vi "RunTest.vi"(8 "error in (no error)":errorcluster, 11 "Prueba01 in":refnum<class "Prueba01.lvclass">) -> (0 "error out":errorcluster, 2 "resultado":string, 3 "Prueba01 out":refnum<class "Prueba01.lvclass">)   [LabVIEW 2019, in "Prueba01.lvclass"]
uses:
  Prueba01.lvclass
  Controles/MessageP01.ctl
  Controles/EstadosP01.ctl
  Prueba01.lvclass/Prueba01.ctl
  RerenceAllControlsToolkit/_get control reference by name.vi
  RerenceAllControlsToolkit/_get mutiple control reference by name.vi
  Instrumento/CNT90/CNT90.lvclass
  Instrumento/Keithley2002/Keithley2002.lvclass
  Instrumento/DS360/DS360.lvclass
panel:
  in  "Tab Control":enum32{"externo", "interno"}(tab)
  out "max_tol_ajuste_ext":dbl format="%.1f"
  out "nivel_ref":dbl
  in  "generar":bool
  out "frec_ref":dbl
  out "cumple":bool
  out "no_cumple":bool
  out "frecuencia":dbl format="%.1f"
  out "nivel":dbl
  in  "señal_antes_ajuste":dbl format="%.1f"
  out "error_ext":dbl
  out "inc_expand_ext":dbl
  in  "seguir_ext":bool
  out "voltaje":dbl
  out "frecuencia 2":dbl
  out "tipo generador":string
  out "max_tol_ajuste_int":dbl
  out "Nivel_interno":dbl
  out "frecuencia_int":dbl
  out "cumple_int":bool
  out "no_cumple_int":bool
  out "frec_ref_int":dbl
  out "nivel_ref_int":dbl
  in  "señal_antes_ajuste_int":dbl
  out "error_ext_int":dbl
  out "inc_extend_int":dbl
  in  "seguir_int":bool
  out "tipo gen_int":string
  # "Elección Señal de Referencia \nsegún marca y modelo de sonómetro"
  # "Cumple"
  # "No Cumple"
  # "Máxima Tolerancia de Ajuste"
  # "Frecuencia"
  # "Nivel"
  # "Frecuencia Señal de Referencia [Hz]"
  # "Nivel de Señal de Referencia [dB] (a)"
  # "Nivel de señal medida antes de ajuste [dB] (b)"
  # "Error [dB]"
  # "Incertidumbre Expandida ± [dB] (k=2)"
  # "1. Indicación a la frecuencia de comprobación. IEC 61672-3: 2006 Cláusula 9"
  # "Monitoreo"
  # "Frecuencia"
  # "Hz"
  # "Voltaje"
  # "V"
  # "Elección Señal de Referencia \nsegún marca y modelo de sonómetro"
  # "Máxima Tolerancia de ajuste"
  # "Cumple"
  # "No Cumple"
  # "Frecuencia"
  # "Nivel"
  # "Frecuencia Señal de Referencia [Hz]"
  # "Nivel de Señal de Referencia [dB] (a)"
  # "Nivel de señal medida antes de ajuste [dB] (b)"
  # "Error [dB]"
  # "Incertidumbre Expandida ± [dB] (k=2)"
  # "1. Indicación a la frecuencia de comprobación. IEC 61672-3: 2006 Cláusula 9"
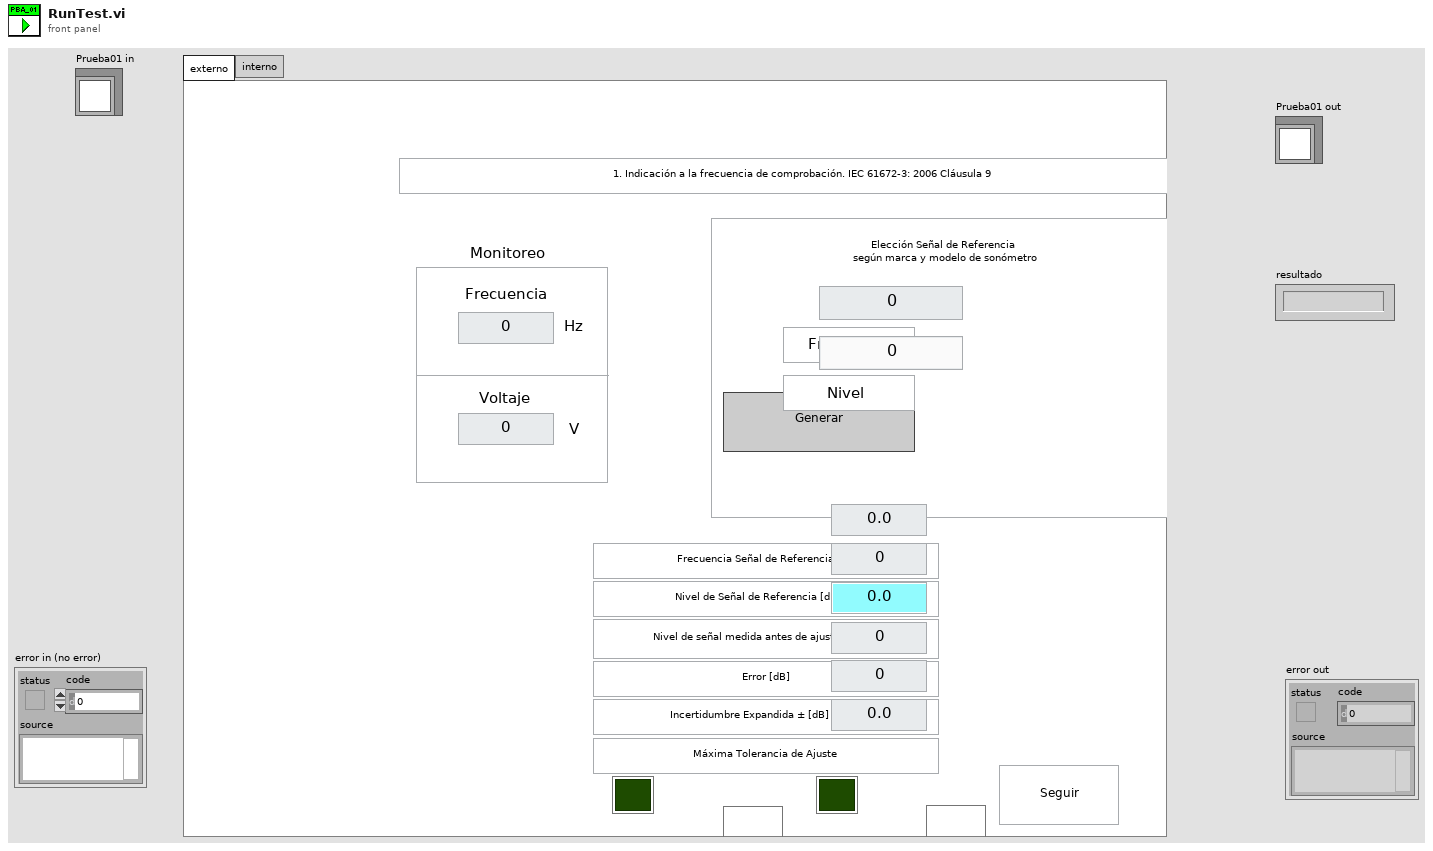
[diagram p1: front panel]
types:
  T1 = typedef "Prueba01.lvclass/EstadosP01.ctl" = enum16{"Inicio", "LeeArchivoConf", "LeeTipoGenerador", "inicio_ext", "inicio_int", "leer_BD", "leer_BD_int", "FrecAmpGEN_ext", "iniciarGEN_ext", "monitoreo", "detenerGEN_ext", "cumplimiento_ext", "cumplimiento_int", "Confirmar Salir", "salir"}
  T2 = typedef "Prueba01.lvclass/MessageP01.ctl" = cluster{"Estados":T1, "Data":variant}
  T3 = enum8{"Enabled", "Disabled", "Disabled and Grayed Out"}
  T4 = cluster{"ControlName":string, "ControlReference":refnum<vi>}[]
  T5 = typedef "Prueba01.lvclass/BD_P01.ctl" = cluster{"frec_ref":dbl, "nivel_presion_ref":dbl, "max_tolerancia_aju":dbl, "inc_expand_ext":dbl, "vol_enviado_CAM":dbl}
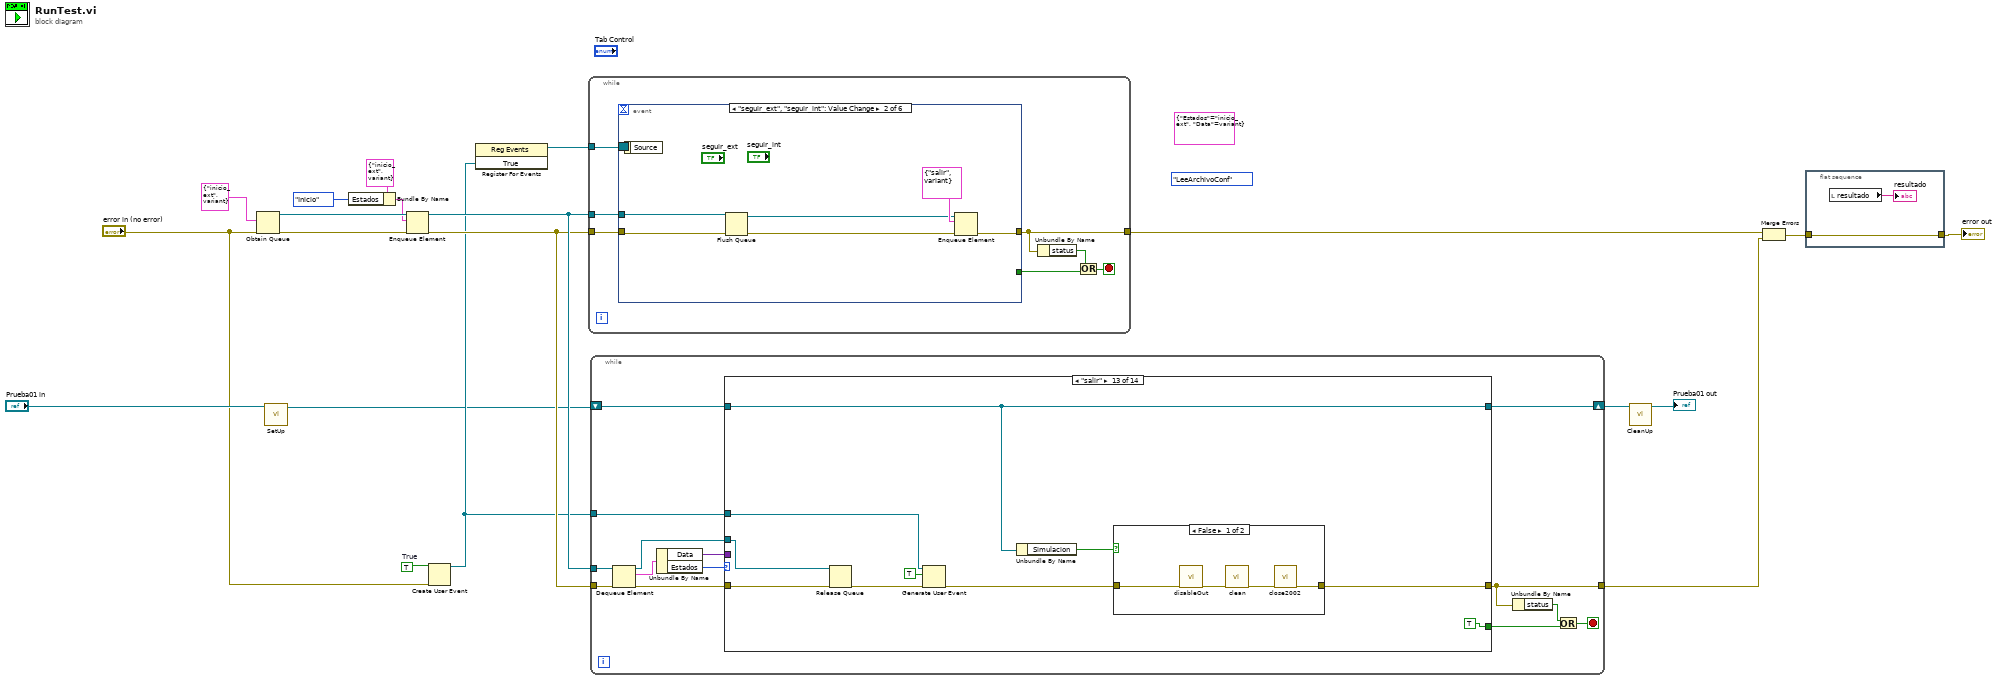
[diagram p0: block diagram]
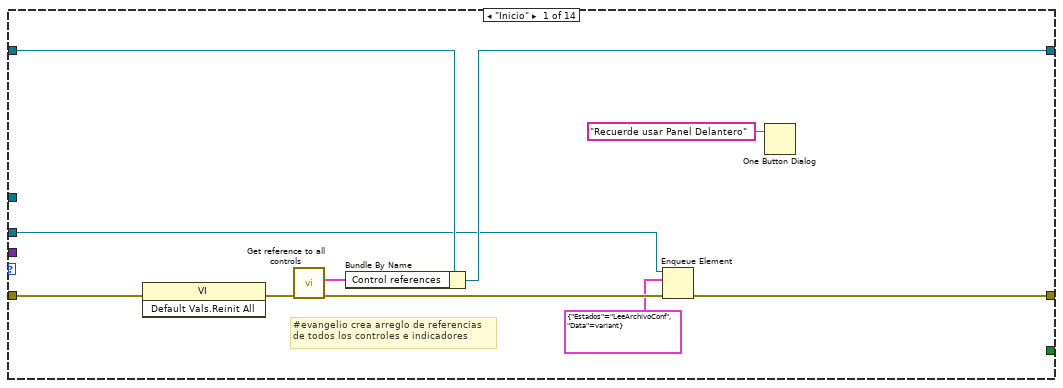
[diagram p2: hidden frame]
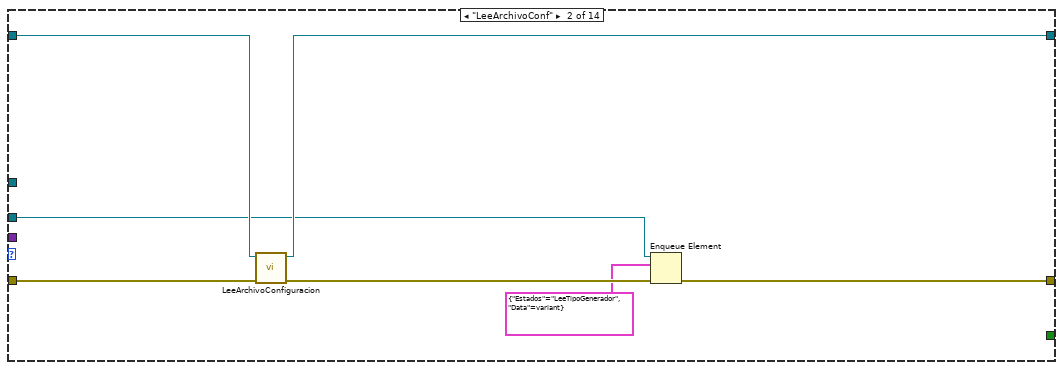
[diagram p3: hidden frame]
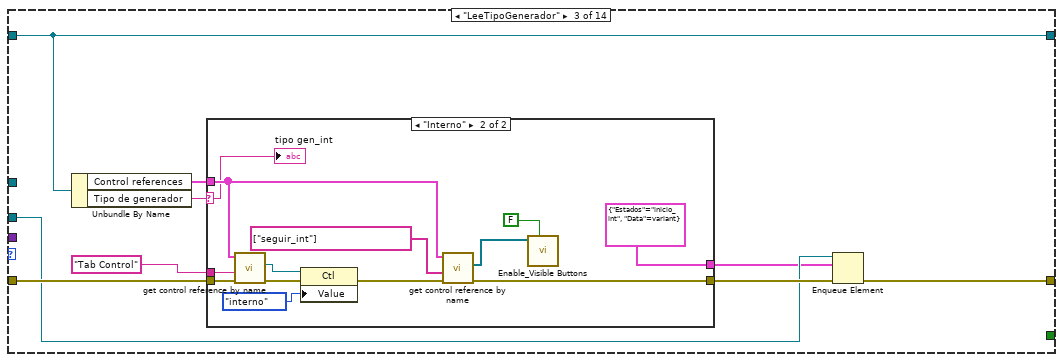
[diagram p4: hidden frame]
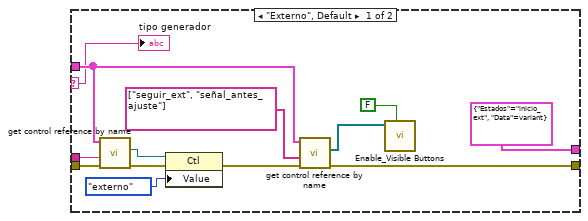
[diagram p5: hidden frame]
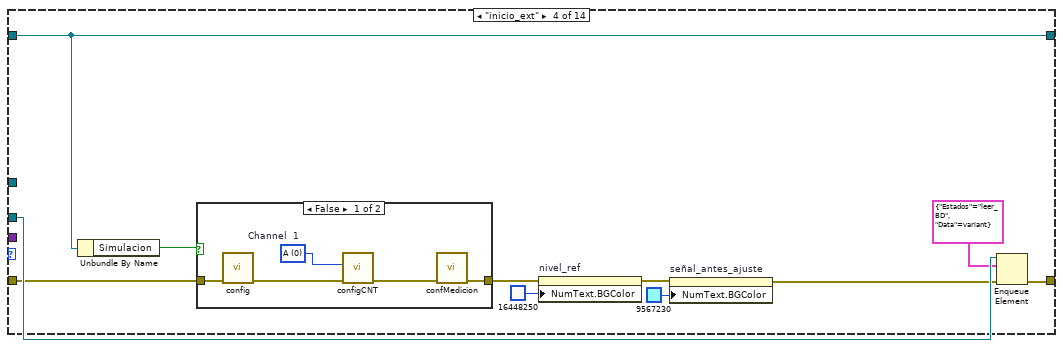
[diagram p6: hidden frame]
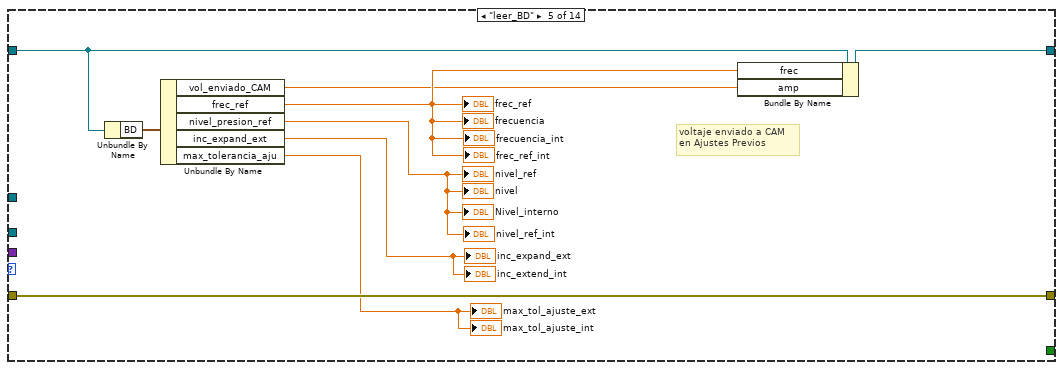
[diagram p8: hidden frame]
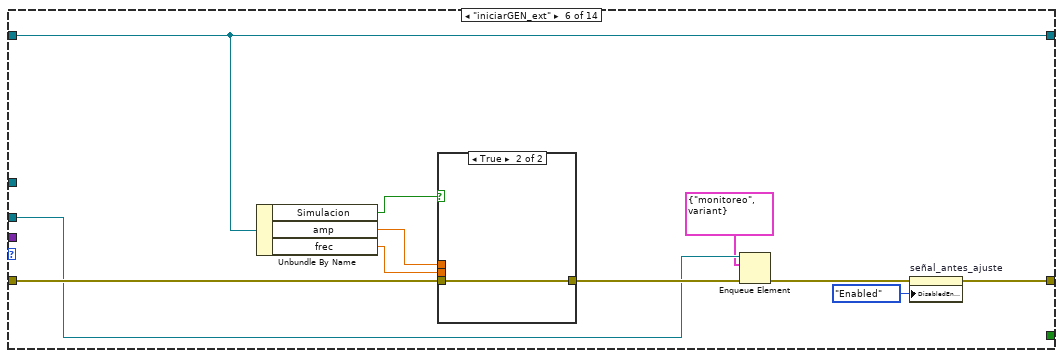
[diagram p9: hidden frame]
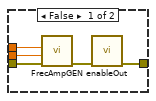
[diagram p10: hidden frame]
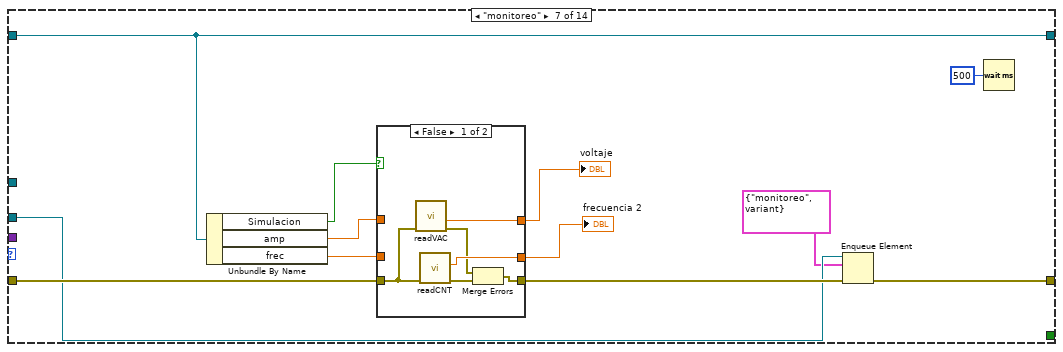
[diagram p11: hidden frame]
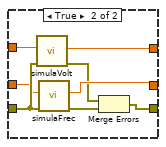
[diagram p12: hidden frame]
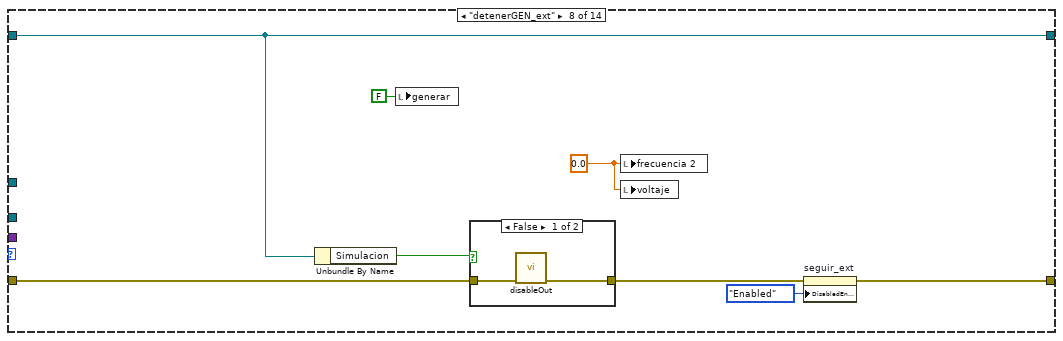
[diagram p13: hidden frame]
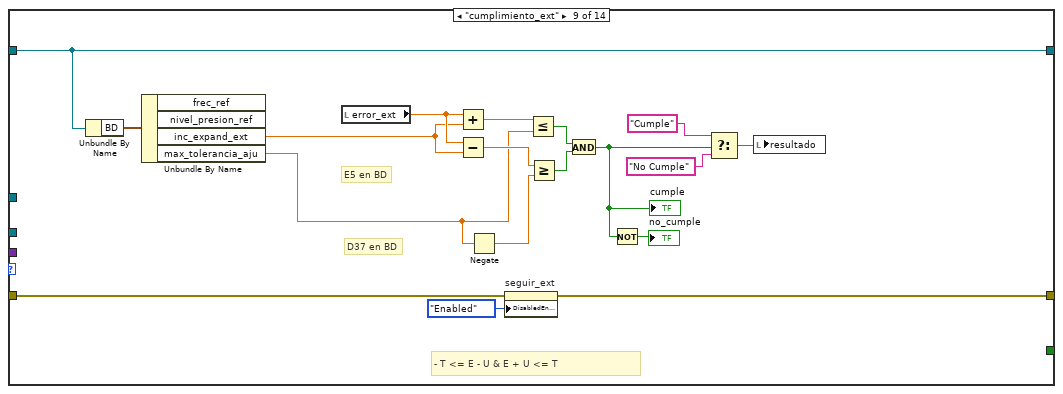
[diagram p15: hidden frame]
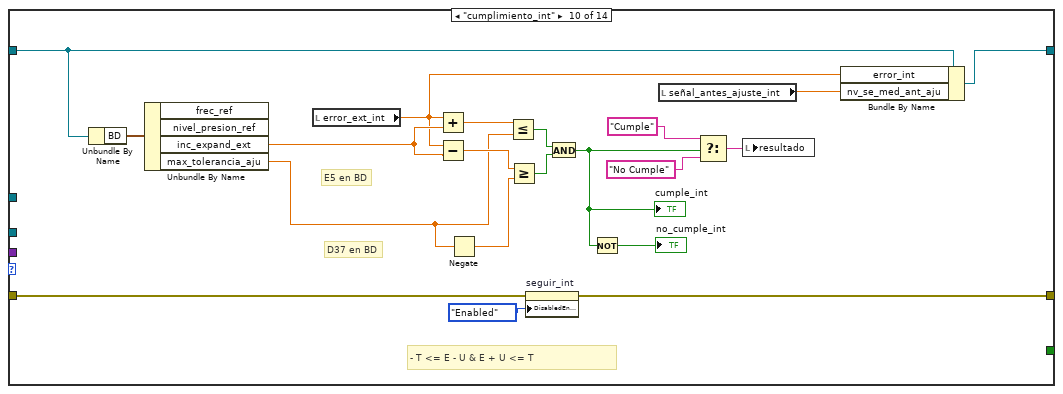
[diagram p16: hidden frame]
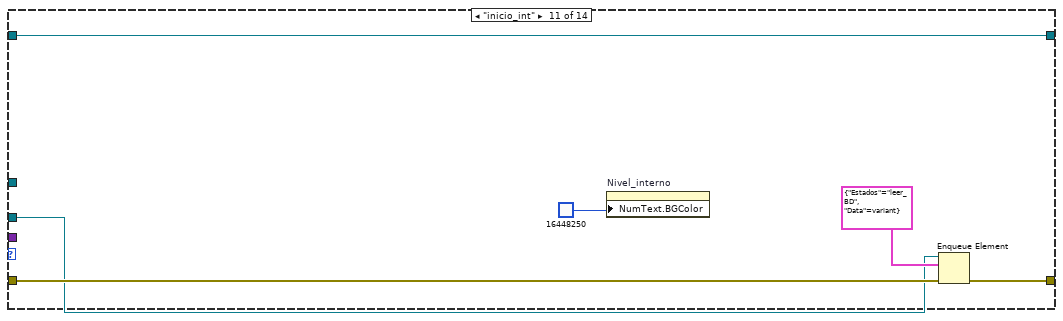
[diagram p17: hidden frame]
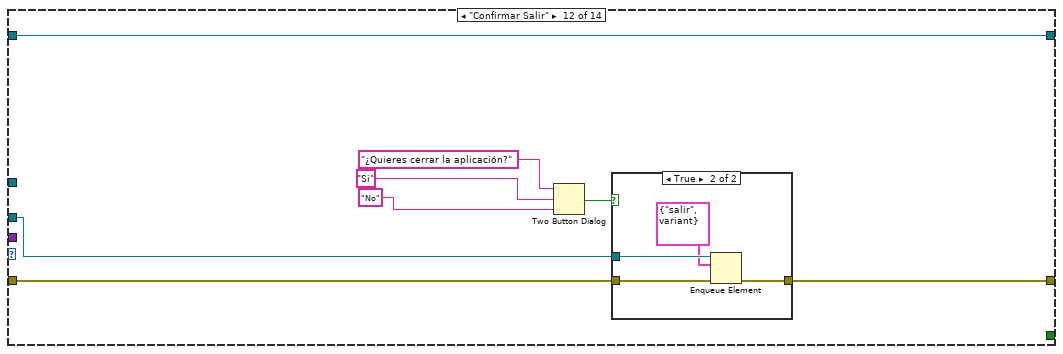
[diagram p18: hidden frame]
diagram:
  w5 = TRUE  # True
  (unwired) EstadosP01."LeeArchivoConf" ("Estados")
  (unwired) T2 {"Estados"=enum."inicio_ext", "Data"=variant}
  n1 = Obtain Queue(element data type=T2 {"Estados"=enum."inicio_ext", "Data"=variant}, error in (no error)="error in (no error)") -> (queue out=w19:refnum<queue>, error out=w18:errorcluster)  [unwired: 3 in, 1 out]
  n2 = call-dynamic "SetUp.vi"("Prueba01 in"="Prueba01 in") -> ("Prueba01 out"=w1:refnum<class "Prueba01.lvclass">)  [unwired: 9 in, 1 out]
  n3 = Bundle By Name(cluster=T2 {"Estados"=enum."inicio_ext", "Data"=variant}, "Estados"=EstadosP01."Inicio") -> (w11:T2)
  n4 = Enqueue Element(queue=w19, element=w11, error in (no error)=w18) -> (queue out=w16:refnum<queue>, error out=w15:errorcluster)  [unwired: 1 in, 1 out]
  n5 = Create User Event(user event datatype=w5, error in="error in (no error)") -> (user event=w2:refnum<user-event>)  [unwired: 1 out]
  n6 = register-events(w2) -> (reference out=w4:refnum<event-registration>)  [unwired: 2 in, 1 out]
  n7 = while {
    tunnel: w16 -> [w26]
    tunnel: w15 -> [w27]
    tunnel: [w24] -> w10
    tunnel: w4 -> [w25]
    stop <- w23 stop-if-true
    n8 = event shown="[1] \"seguir_ext\", \"seguir_int\": Value Change" {
      selector: w25 -> [_ _ _ _ _ _]
      dyn-events: _ -> [_ _ _ _ _ _]
      timeout: _ -> [_ _ _ _ _ _]
      tunnel: w27 -> [w31 w40 w41 w51 w57 w64]
      tunnel: w26 -> [w28 w36 _ w44 w54 w65]
      tunnel: [w30 w39 w41 w50 w55 w63] -> w24
      tunnel: [_ _ TRUE _ _ _] -> w21
      event "señal_antes_ajuste": Value Change {
        n9 = event-data() -> ("NewVal"=w33:dbl)  [unwired: 1 in]
        n10 = local read "nivel"() -> (w32:dbl)
        n11 = Subtract(x=w33, y=w32) -> (x-y=→"error_ext":dbl)
        n12 = Enqueue Element(queue=w28, element=T2 {"Estados"=enum."cumplimiento_ext", "Data"=variant}, error in (no error)=w31) -> (error out=w30:errorcluster)  [unwired: 1 in, 2 out]
      }
      event "seguir_ext", "seguir_int": Value Change {
        n13 = event-data() -> ()  [unwired: 1 in, 1 out]
        n14 = Flush Queue(queue=w36, error in (no error)=w40) -> (queue out=w35:refnum<queue>, error out=w37:errorcluster)  [unwired: 1 out]
        n15 = Enqueue Element(queue=w35, element=T2 {"Estados"=enum."salir", "Data"=variant}, error in (no error)=w37) -> (error out=w39:errorcluster)  [unwired: 1 in, 2 out]
      }
      event User Event {
        n16 = event-data() -> ()  [unwired: 1 in, 5 out]
      }
      event "generar": Value Change {
        n17 = event-data() -> ("NewVal"=w48:bool)  [unwired: 1 in]
        n18 = Flush Queue(queue=w44, error in (no error)=w51) -> (queue out=w43:refnum<queue>, error out=w45:errorcluster)  [unwired: 1 out]
        n19 = Equal?(x=w48, y=TRUE) -> (x = y?=w46:bool)
        n20 = case shown="True" w46 {
          tunnel: [T2 {"Estados"=enum."detenerGEN_ext", "Data"=variant} ("element") T2 {"Estados"=enum."iniciarGEN_ext", "Data"=variant} ("element")] -> w49
          frame False {
          }
          frame True {
          }
        }
        n21 = Enqueue Element(queue=w43, element=w49, error in (no error)=w45) -> (error out=w50:errorcluster)  [unwired: 1 in, 2 out]
      }
      event "señal_antes_ajuste_int": Value Change {
        n22 = event-data() -> ("NewVal"=w58:dbl)  [unwired: 1 in]
        n23 = local read "nivel_ref_int"() -> (w59:dbl)
        n24 = Subtract(x=w58, y=w59) -> (x-y=→"error_ext_int":dbl)
        n25 = Enqueue Element(queue=w54, element=T2 {"Estados"=enum."cumplimiento_int", "Data"=variant}, error in (no error)=w57) -> (error out=w55:errorcluster)  [unwired: 1 in, 2 out]
      }
      event Panel Close? {
        n26 = event-data() -> ()  [unwired: 1 in, 1 out]
        n27 = Enqueue Element(queue=w65, element=T2 {"Estados"=enum."Confirmar Salir", "Data"=variant}, error in (no error)=w64) -> (error out=w63:errorcluster)  [unwired: 1 in, 2 out]
        n28 = event-data("Discard?"=TRUE) -> ()  [unwired: 1 in, 1 out]
      }
    }
    n29 = Unbundle By Name(w24) -> ("status"=w22:bool)
    n30 = Or(x=w22, y=w21) -> (x .or. y?=w23:bool)
  }
  n31 = while {
    tunnel: w16 -> [w79]
    tunnel: w15 -> [w78]
    tunnel: [w68] -> w9
    shift-right: [w67] -> w14
    shift-left: w1 -> [w69]
    tunnel: w2 -> [w66]
    stop <- w72 stop-if-true
    n32 = Dequeue Element(queue=w79, error in (no error)=w78) -> (queue out=w76:refnum<queue>, element=w77:T2, error out=w73:errorcluster)  [unwired: 1 in, 1 out]
    n33 = Unbundle By Name(w77) -> ("Data"=w74:variant, "Estados"=w75:T1)
    n34 = case shown="\"salir\"" w75 {
      tunnel: w76 -> [w82 w91 w98 w138 _ w162 w183 _ _ _ w250 w257 w277 _]
      tunnel: w74 -> [_ _ _ _ _ _ _ _ _ _ _ _ _ _]
      tunnel: w73 -> [w87 w96 w102 w136 w157 w168 w185 w208 w229 w235 w252 w259 w278 w285]
      tunnel: [w83 w92 w99 w139 w157 w159 w186 w202 w213 w234 w251 w258 w274 w285] -> w68
      tunnel: [_ _ _ _ _ _ _ _ _ _ _ _ TRUE _] -> w70
      tunnel: w69 -> [w85 w95 w100 w133 w155 w166 w180 w204 w216 w233 w255 w263 w273 w284]
      tunnel: [w84 w94 w100 w133 w156 w166 w180 w204 w216 w232 w255 w263 w273 w284] -> w67
      tunnel: w66 -> [_ _ _ _ _ _ _ _ _ _ _ _ w270 _]
      frame "Inicio" {
        # "#evangelio crea arreglo de referencias\nde todos los controles e indicadores"
        n35 = invoke class="VI" method="Default Vals.Reinit All"(error in=w87) -> (error out=w89:errorcluster)  [unwired: 2 in, 2 out]
        n36 = call "Get reference to all controls.vi"("error in (no error)"=w89) -> ("error out"=w86:errorcluster, "Control references"=w88:T4)  [unwired: 5 in]
        n37 = Bundle By Name(cluster=w85, "Control references"=w88) -> (w84:refnum<class "Prueba01.lvclass">)
        n38 = Enqueue Element(queue=w82, element=T2 {"Estados"=enum."LeeArchivoConf", "Data"=variant}, error in (no error)=w86) -> (error out=w83:errorcluster)  [unwired: 1 in, 2 out]
        n39 = One Button Dialog(message="Recuerde usar Panel Delantero") -> ()  [unwired: 1 in, 1 out]
      }
      frame "LeeArchivoConf" {
        n40 = call "LeeArchivoConfiguracion.vi"("error in (no error)"=w96, "Prueba01 in"=w95) -> ("error out"=w93:errorcluster, "Prueba01 out"=w94:refnum<class "Prueba01.lvclass">)  [unwired: 8 in]
        n41 = Enqueue Element(queue=w91, element=T2 {"Estados"=enum."LeeTipoGenerador", "Data"=variant}, error in (no error)=w93) -> (error out=w92:errorcluster)  [unwired: 1 in, 2 out]
      }
      frame "LeeTipoGenerador" {
        n42 = Unbundle By Name(w100) -> ("Control references"=w104:T4, "Tipo de generador"=w105:string)
        n43 = case shown="\"Interno\"" w105 {
          selector: w105 -> [w109 w122]
          tunnel: w102 -> [w118 w131]
          tunnel: w104 -> [w113 w126]
          tunnel: "Tab Control" -> [w117 w130]
          tunnel: [w111 w124] -> w101
          tunnel: [T2 {"Estados"=enum."inicio_ext", "Data"=variant} ("element") T2 {"Estados"=enum."inicio_int", "Data"=variant} ("element")] -> w97
          frame "Externo", Default {
            n44 = call-poly "get control reference by name.vi"("error in (no error)"=w118, "Control name"=w117, "Control references"=w113) -> ("error out"=w115:errorcluster, "Ctl Refnum"=w116:refnum<vi>)  [unwired: 3 in]
            n45 = property class="Ctl"(reference=w116, error in=w115, "Value"=enum32{"externo", "interno"}."externo" ("Tab Control")) -> (error out=w112:errorcluster)  [unwired: 1 out]
            n46 = call-poly "get control reference by name.vi"("error in (no error)"=w112, "Control names"=string[] ["seguir_ext", "señal_antes_ajuste"], "Control references"=w113) -> ("error out"=w111:errorcluster, "References"=w106:refnum<vi>[])  [unwired: 3 in]
            n47 = call "Enable_Visible Buttons.vi"("Enable? (T)"=FALSE, "Controls Ref Array"=w106) -> ()  [unwired: 10 in]
            "tipo generador" <- w109
          }
          frame "Interno" {
            n48 = call-poly "get control reference by name.vi"("error in (no error)"=w131, "Control name"=w130, "Control references"=w126) -> ("error out"=w128:errorcluster, "Ctl Refnum"=w129:refnum<vi>)  [unwired: 3 in]
            n49 = property class="Ctl"(reference=w129, error in=w128, "Value"=enum32{"externo", "interno"}."interno" ("Tab Control")) -> (error out=w125:errorcluster)  [unwired: 1 out]
            n50 = call-poly "get control reference by name.vi"("error in (no error)"=w125, "Control names"=string[] ["seguir_int"], "Control references"=w126) -> ("error out"=w124:errorcluster, "References"=w119:refnum<vi>[])  [unwired: 3 in]
            n51 = call "Enable_Visible Buttons.vi"("Enable? (T)"=FALSE, "Controls Ref Array"=w119) -> ()  [unwired: 10 in]
            "tipo gen_int" <- w122
          }
        }
        n52 = Enqueue Element(queue=w98, element=w97, error in (no error)=w101) -> (error out=w99:errorcluster)  [unwired: 1 in, 2 out]
      }
      frame "inicio_ext" {
        n53 = Unbundle By Name(w133) -> ("Simulacion"=w132:bool)
        n54 = case shown="False" w132 {
          tunnel: w136 -> [w146 w148]
          tunnel: [w143 w148] -> w135
          frame False {
            w145 = 0 items=["A", "B"]  # Channel  1
            n55 = call "config.vi"("error in (no error)"=w146) -> ("error out"=w147:errorcluster)  [unwired: 9 in, 1 out]
            n56 = call "configCNT.vi"("error in (no error)"=w147, "Channel  1"=w145) -> ("error out"=w144:errorcluster)  [unwired: 8 in, 1 out]
            n57 = call "confMedicion.vi"("error in (no error)"=w144) -> ("error out"=w143:errorcluster)  [unwired: 9 in, 1 out]
          }
          frame True {
          }
        }
        n58 = property on="nivel_ref" class="DigNum (strict)"(error in=w135, "NumText.BGColor"=u32 16448250) -> (error out=w142:errorcluster)  [unwired: 1 in, 1 out]
        n59 = property on="señal_antes_ajuste" class="DigNum (strict)"(error in=w142, "NumText.BGColor"=u32 9567230) -> (error out=w134:errorcluster)  [unwired: 1 in, 1 out]
        n60 = Enqueue Element(queue=w138, element=T2 {"Estados"=enum."leer_BD", "Data"=variant}, error in (no error)=w134) -> (error out=w139:errorcluster)  [unwired: 1 in, 2 out]
      }
      frame "leer_BD" {
        # "voltaje enviado a CAM\nen Ajustes Previos"
        n61 = Unbundle By Name(w155) -> ("BD"=w154:T5)
        n62 = Unbundle By Name(w154) -> ("vol_enviado_CAM"=w150:dbl, "frec_ref"=w151:dbl, "nivel_presion_ref"=→"nivel_ref" →"nivel" →"Nivel_interno" →"nivel_ref_int":dbl, "inc_expand_ext"=→"inc_expand_ext" →"inc_extend_int":dbl, "max_tolerancia_aju"=→"max_tol_ajuste_ext" →"max_tol_ajuste_int":dbl)
        "frec_ref" <- w151
        "frecuencia" <- w151
        "frecuencia_int" <- w151
        "frec_ref_int" <- w151
        n63 = Bundle By Name(cluster=w155, "frec"=w151, "amp"=w150) -> (w156:refnum<class "Prueba01.lvclass">)
      }
      frame "iniciarGEN_ext" {
        n64 = Unbundle By Name(w166) -> ("Simulacion"=w160:bool, "amp"=w165:dbl, "frec"=w164:dbl)
        n65 = case shown="True" w160 {
          tunnel: w168 -> [w172 w174]
          tunnel: [w171 w174] -> w167
          tunnel: w165 -> [w170 _]
          tunnel: w164 -> [w169 _]
          frame False {
            n66 = call "FrecAmpGEN.vi"("error in (no error)"=w172, "Frec (Hz)"=w169, "Amplitud (Vrms)"=w170) -> ("error out"=w173:errorcluster)  [unwired: 7 in, 1 out]
            n67 = call "enableOut.vi"("error in (no error)"=w173) -> ("error out"=w171:errorcluster)  [unwired: 9 in, 1 out]
          }
          frame True {
          }
        }
        n68 = Enqueue Element(queue=w162, element=T2 {"Estados"=enum."monitoreo", "Data"=variant}, error in (no error)=w167) -> (error out=w163:errorcluster)  [unwired: 1 in, 2 out]
        n69 = property on="señal_antes_ajuste" class="DigNum (strict)"(error in=w163, "DisabledEnum"=T3."Enabled" ("Disabled")) -> (error out=w159:errorcluster)  [unwired: 1 in, 1 out]
      }
      frame "monitoreo" {
        n70 = Unbundle By Name(w180) -> ("Simulacion"=w175:bool, "amp"=w178:dbl, "frec"=w179:dbl)
        n71 = case shown="False" w175 {
          tunnel: w185 -> [w189 w196]
          tunnel: [w188 w195] -> w184
          tunnel: [w191 w199] -> w181
          tunnel: w179 -> [_ w193]
          tunnel: w178 -> [_ w198]
          tunnel: [w190 w197] -> w176
          frame False {
            n72 = call "readVAC.vi"("error in (no error)"=w189) -> ("error out"=w187:errorcluster, "medicion"=w191:dbl)  [unwired: 7 in, 2 out]
            n73 = call "readCNT.vi"("error in (no error)"=w189) -> ("error out"=w192:errorcluster, "medicion"=w190:dbl)  [unwired: 8 in, 1 out]
            n74 = Merge Errors(w187, w192) -> (w188:errorcluster)
          }
          frame True {
            n75 = call "simulaVolt.vi"("error in (no error)"=w196, "volt in"=w198) -> ("error out"=w194:errorcluster, "volt out"=w199:dbl)  [unwired: 7 in, 1 out]
            n76 = call "simulaFrec.vi"("error in (no error)"=w196, "frec in"=w193) -> ("error out"=w200:errorcluster, "frec out"=w197:dbl)  [unwired: 7 in, 1 out]
            n77 = Merge Errors(w194, w200) -> (w195:errorcluster)
          }
        }
        "frecuencia 2" <- w176
        "voltaje" <- w181
        n78 = Enqueue Element(queue=w183, element=T2 {"Estados"=enum."monitoreo", "Data"=variant}, error in (no error)=w184) -> (error out=w186:errorcluster)  [unwired: 1 in, 2 out]
        n79 = Wait (ms)(milliseconds to wait=u32 500) -> ()  [unwired: 1 out]
      }
      frame "detenerGEN_ext" {
        w206 = 0.0 ("frecuencia 2")
        n80 = Unbundle By Name(w204) -> ("Simulacion"=w203:bool)
        n81 = local write "generar"(FALSE ("generar")) -> ()
        n82 = case shown="False" w203 {
          tunnel: w208 -> [w210 w211]
          tunnel: [w209 w211] -> w207
          frame False {
            n83 = call "disableOut.vi"("error in (no error)"=w210) -> ("error out"=w209:errorcluster)  [unwired: 9 in, 1 out]
          }
          frame True {
          }
        }
        n84 = local write "frecuencia 2"(w206) -> ()
        n85 = local write "voltaje"(w206) -> ()
        n86 = property on="seguir_ext" class="Bool"(error in=w207, "DisabledEnum"=T3."Enabled" ("Disabled")) -> (error out=w202:errorcluster)  [unwired: 1 in, 1 out]
      }
      frame "cumplimiento_ext" {
        # "- T <= E - U & E + U <= T"
        # "D37 en BD"
        # "E5 en BD"
        n87 = Unbundle By Name(w216) -> ("BD"=w217:T5)
        n88 = Unbundle By Name(w217) -> ("inc_expand_ext"=w215:dbl, "max_tolerancia_aju"=w214:dbl)  [unwired: 2 out]
        n89 = local read "error_ext"() -> (w227:dbl)
        n90 = Add(x=w227, y=w215) -> (x+y=w226:dbl)
        n91 = Subtract(x=w227, y=w215) -> (x-y=w223:dbl)
        n92 = Negate(x=w214) -> (-x=w221:dbl)
        n93 = property on="seguir_ext" class="Bool"(error in=w229, "DisabledEnum"=T3."Enabled" ("Disabled")) -> (error out=w213:errorcluster)  [unwired: 1 in, 1 out]
        n94 = Less Or Equal?(x=w226, y=w214) -> (x <= y?=w225:bool)
        n95 = Greater Or Equal?(x=w223, y=w221) -> (x >= y?=w224:bool)
        n96 = And(x=w225, y=w224) -> (x .and. y?=w222:bool)
        "cumple" <- w222
        n97 = Not(x=w222) -> (.not. x?=→"no_cumple":bool)
        n98 = Select(t="Cumple", s=w222, f="No Cumple") -> (s? t:f=w220:string)
        n99 = local write "resultado"(w220) -> ()
      }
      frame "cumplimiento_int" {
        # "D37 en BD"
        # "E5 en BD"
        # "- T <= E - U & E + U <= T"
        n100 = Unbundle By Name(w233) -> ("BD"=w239:T5)
        n101 = Unbundle By Name(w239) -> ("inc_expand_ext"=w238:dbl, "max_tolerancia_aju"=w237:dbl)  [unwired: 2 out]
        n102 = local read "error_ext_int"() -> (w231:dbl)
        n103 = Add(x=w231, y=w238) -> (x+y=w249:dbl)
        n104 = Subtract(x=w231, y=w238) -> (x-y=w246:dbl)
        n105 = Negate(x=w237) -> (-x=w245:dbl)
        n106 = Less Or Equal?(x=w249, y=w237) -> (x <= y?=w248:bool)
        n107 = Greater Or Equal?(x=w246, y=w245) -> (x >= y?=w247:bool)
        n108 = property on="seguir_int" class="Bool"(error in=w235, "DisabledEnum"=T3."Enabled" ("Disabled")) -> (error out=w234:errorcluster)  [unwired: 1 in, 1 out]
        n109 = And(x=w248, y=w247) -> (x .and. y?=w243:bool)
        "cumple_int" <- w243
        n110 = Not(x=w243) -> (.not. x?=→"no_cumple_int":bool)
        n111 = local read "señal_antes_ajuste_int"() -> (w230:dbl)
        n112 = Select(t="Cumple", s=w243, f="No Cumple") -> (s? t:f=w244:string)
        n113 = local write "resultado"(w244) -> ()
        n114 = Bundle By Name(cluster=w233, "error_int"=w231, "nv_se_med_ant_aju"=w230) -> (w232:refnum<class "Prueba01.lvclass">)
      }
      frame "inicio_int" {
        n115 = property on="Nivel_interno" class="DigNum (strict)"("NumText.BGColor"=u32 16448250) -> ()  [unwired: 2 in, 2 out]
        n116 = Enqueue Element(queue=w250, element=T2 {"Estados"=enum."leer_BD", "Data"=variant}, error in (no error)=w252) -> (error out=w251:errorcluster)  [unwired: 1 in, 2 out]
      }
      frame "Confirmar Salir" {
        n117 = Two Button Dialog(message="¿Quieres cerrar la aplicación?", 1:"No" ("T button name (\"OK\")"), 2:"Si" ("T button name (\"OK\")")) -> (T button?=w256:bool)
        n118 = case shown="True" w256 {
          tunnel: w259 -> [w264 w268]
          tunnel: [w264 w267] -> w258
          tunnel: w257 -> [_ w266]
          frame False {
          }
          frame True {
            n119 = Enqueue Element(queue=w266, element=T2 {"Estados"=enum."salir", "Data"=variant}, error in (no error)=w268) -> (error out=w267:errorcluster)  [unwired: 1 in, 2 out]
          }
        }
      }
      frame "salir" {
        n120 = Release Queue(queue=w277, error in (no error)=w278) -> (error out=w276:errorcluster)  [unwired: 1 in, 2 out]
        n121 = Generate User Event(user event=w270, event data cluster=TRUE ("event data"), error in=w276) -> (error out=w271:errorcluster)  [unwired: 1 in, 1 out]
        n122 = Unbundle By Name(w273) -> ("Simulacion"=w272:bool)
        n123 = case shown="False" w272 {
          tunnel: w271 -> [w282 w283]
          tunnel: [w279 w283] -> w274
          frame False {
            n124 = call "disableOut.vi"("error in (no error)"=w282) -> ("error out"=w281:errorcluster)  [unwired: 9 in, 1 out]
            n125 = call "clean.vi"("error in (no error)"=w281) -> ("error out"=w280:errorcluster)  [unwired: 9 in, 1 out]
            n126 = call "close2002.vi"("error in (no error)"=w280) -> ("error out"=w279:errorcluster)  [unwired: 9 in, 1 out]
          }
          frame True {
          }
        }
      }
      frame Default {
      }
    }
    n127 = Unbundle By Name(w68) -> ("status"=w71:bool)
    n128 = Or(x=w71, y=w70) -> (x .or. y?=w72:bool)
  }
  n129 = call-dynamic "CleanUp.vi"("Prueba01 in"=w14) -> ("Prueba01 out"=→"Prueba01 out":refnum<class "Prueba01.lvclass">)  [unwired: 9 in, 1 out]
  n130 = Merge Errors(w10, w9) -> (w8:errorcluster)
  n131 = flat-sequence {
    tunnel: w8 -> [w286]
    tunnel: [w286] -> w7
    frame #0 {
      n132 = local read "resultado"() -> (→"resultado":string)
    }
  }
  "error out" <- w7
